vi "start galvo task.vi"(8 "error in (no error)":errorcluster, 11 "Waveform in":refnum<class "Waveform.lvclass">) -> (0 "error out":errorcluster, 3 "Waveform out":refnum<class "Waveform.lvclass">)   [LabVIEW 2012, in "Waveform.lvclass"]
uses:
  Waveform.lvclass
  Waveform.lvclass/Waveform.ctl
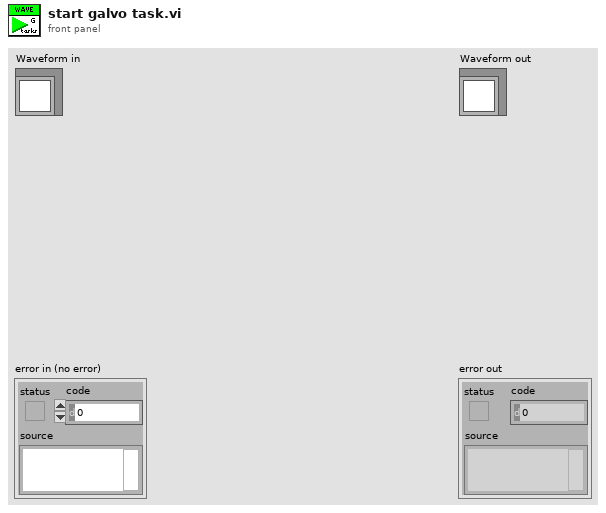
[diagram p1: front panel]
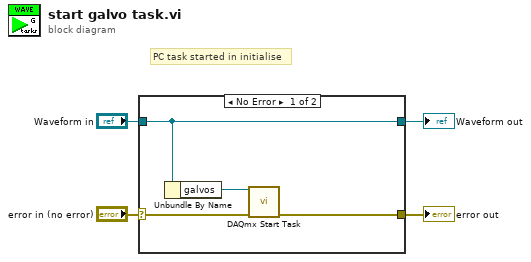
[diagram p0: block diagram]
diagram:
  # "PC task started in initialise"
  n1 = case shown="No Error" "error in (no error)" {
    selector: "error in (no error)" -> [w8 w10]
    tunnel: [w5 w10] -> w3
    tunnel: [w7 w9] -> w1
    tunnel: "Waveform in" -> [w7 w9]
    frame No Error {
      n2 = Unbundle By Name(w7) -> ("galvos"=w6:refnum<k21>)
      n3 = call <vilib>:"DAQmx Start Task.vi"("task/channels in"=w6, "error in"=w8) -> ("error out"=w5:errorcluster)  [unwired: 12 in, 1 out]
    }
    frame Error {
    }
  }
  "error out" <- w3
  "Waveform out" <- w1
